vi "FTW-JSON-Destroy.vi"(0 "JSON Object":refnum<data-value>, 11 "error in":errorcluster) -> (15 "error out":errorcluster)   [LabVIEW 2014]
uses:
  core/FTW-JSON-Core-Structure.ctl
  error/FTW-ERR-ThrowGenericError.vi
  error/FTW-ERR-ThrowError.vi
  error/FTW-ERR-CallChain.vi
  string/FTW-STR-ReplaceWhitespace.vi
panel:
  # "Inputs"
  # "Outputs"
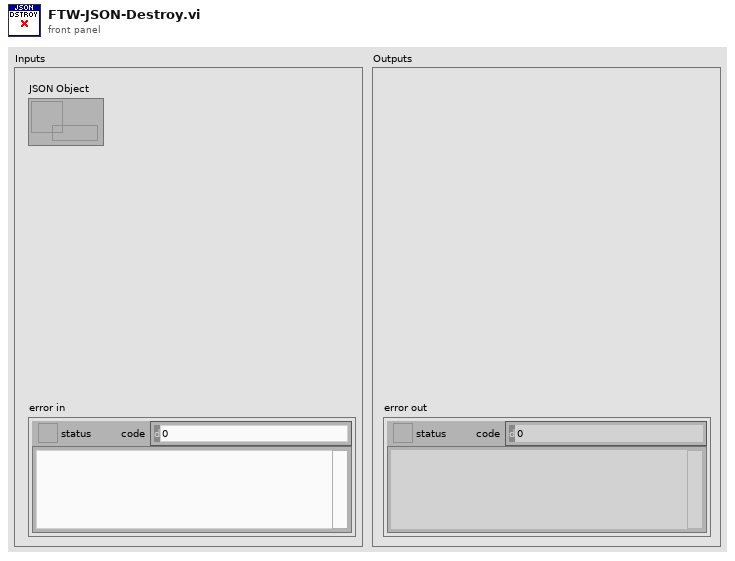
[diagram p1: front panel]
types:
  T1 = typedef "FTW-JSON-Core-Structure.ctl" = cluster{"JSON Object":i64, "Encoding Flags":i64, "Decoding Flags":i64}
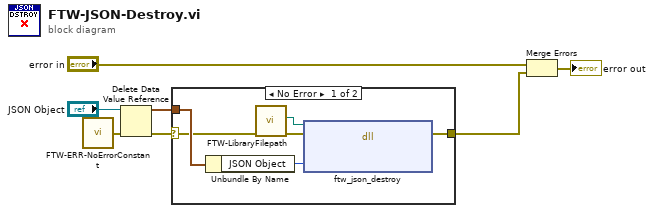
[diagram p0: block diagram]
diagram:
  n1 = call "FTW-ERR-NoErrorConstant.vi"() -> ("no error"=w1:errorcluster)
  n2 = Delete Data Value Reference(data value reference="JSON Object", error in=w1) -> (data value=w3:T1, error out=w2:errorcluster)
  n3 = case shown="No Error" w2 {
    selector: w2 -> [w8 w14]
    tunnel: [w11 w14] -> w6
    tunnel: w3 -> [w10 _]
    frame No Error {
      n4 = Unbundle By Name(w10) -> ("JSON Object"=w9:i64)
      n5 = call "FTW-LibraryFilepath.vi"("error in"=w8) -> ("error out"=w13:errorcluster, "Library Filepath"=w12:path)  [unwired: 8 in, 1 out]
      n6 = dll-call lib="?" fn="ftw_json_destroy"(path in=w12, error in=w13, "JSON Object Pointer"=w9) -> (error out=w11:errorcluster)  [unwired: 3 in, 1 out]
    }
    frame Error {
    }
  }
  n7 = Merge Errors("error in", w6) -> (→"error out":errorcluster)
